vi "Subtask1_Rotate.vi"   [LabVIEW 2016]
uses:
  <vilib>/NXT/Block Support/NXT_InputPort.ctl
  <vilib>/NXT/Block Support/NXT_OutputPort.ctl
  <vilib>/NXT/Dual Mode Library/Sensors/EV3_Gyro_Angle.vi
  <vilib>/NXT/Dual Mode Library/Waits/Wait_Num.vi
  <vilib>/NXT/NXTIO Xnodes/NXTIONodeSubVIs/NXTMoveMotors.vi
  <vilib>/NXT/Subs/LVHSConnector.ctl
  <vilib>/NXT/NXTIO Xnodes/AddressXNode/NXTIOAddress.xnode
  <vilib>/NXT/NXTIO Xnodes/NXTIOXNode/NXTIO.xnode
  <vilib>/NXT/LegoClasses/BrickReference/BrickReference.lvclass
types:
  T1 = typedef "LVHSConnector.ctl" = refnum<class "BrickReference.lvclass">
  T2 = typedef "NXT_InputPort.ctl" = u32
  T3 = typedef "NXT_OutputPort.ctl" = u8
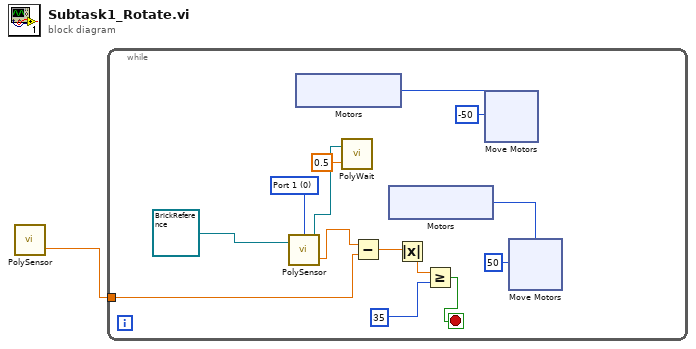
[diagram p0: block diagram]
diagram:
  n1 = call-poly <vilib>:"PolySensor.vi"() -> ("Degrees"=w1:sgl)  [unwired: 3 in, 1 out]
  n2 = while {
    tunnel: w1 -> [w5]
    stop <- w7 stop-if-true
    w15 = T2 0 items=["Port 1", "Port 2", "Port 3", "Port 4"] ("Port (Port 1)")
    n3 = call-poly <vilib>:"PolySensor.vi"("NXT/EV3"=T1 refnum, "Port (Port 1)"=w15) -> ("Degrees"=w6:sgl, "NXT/EV3"=w4:T1)  [unwired: 1 in]
    n4 = xnode "Motors"() -> ("Motor"=w14:T3)
    n5 = call-poly <vilib>:"PolyWait.vi"("Time (1 sec)"=sgl 0.5, "NXT/EV3"=w4) -> ()  [unwired: 2 in, 1 out]
    n6 = Subtract(x=w6, y=w5) -> (x-y=w9:sgl)
    n7 = xnode "Motors"() -> ("Motor"=w13:T3)
    n8 = Absolute Value(x=w9) -> (abs(x)=w8:sgl)
    n9 = Greater Or Equal?(x=w8, y=35) -> (x >= y?=w7:bool)
    n10 = xnode "Move Motors"("Power/Speed 1"=i8 -50, "Motors"=w14) -> ()  [unwired: 1 in, 1 out]
    n11 = xnode "Move Motors"("Power/Speed 1"=i8 50, "Motors"=w13) -> ()  [unwired: 1 in, 1 out]
  }
